vi "7.vi"() -> ()   [LabVIEW 2017]
uses:
  <vilib>/Waveform/WDTFileIO.llb/ Write Waveform to File.vi
  <vilib>/Waveform/WDTFileIO.llb/Read Waveform from File.vi
  <vilib>/Analysis/NI_AALBase.lvlib
panel:
  out "数组":dbl[](array[numeric])
  out "波形图":waveform(dbl)(graph)
  in  "cycles":dbl=1.0 caption="周期" format="%0.2f"
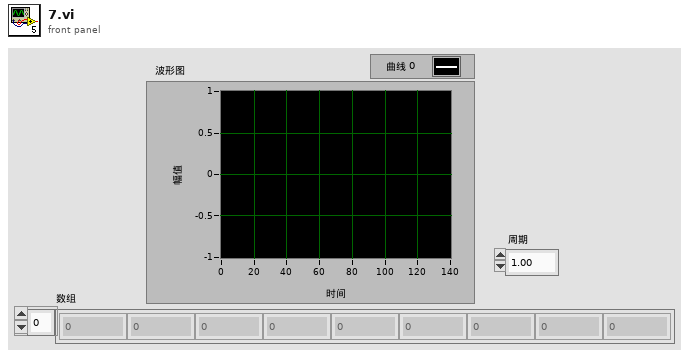
[diagram p1: front panel]
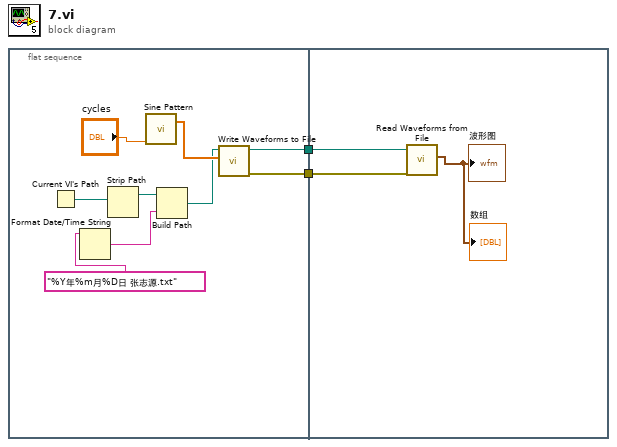
[diagram p0: block diagram]
diagram:
  n1 = flat-sequence {
    tunnel: [w4] -> w2
    tunnel: [w3] -> w1
    tunnel: w2 -> [w14]
    tunnel: w1 -> [w13]
    frame #0 {
      n2 = Current VI's Path() -> (path=w10:path)
      n3 = Format Date/Time String(time format string (%c)="%Y年%m月%D日 张志源.txt" ("时间格式字符串(%c)")) -> (date/time string=w8:string)  [unwired: 2 in]
      n4 = Strip Path(path=w10) -> (stripped path=w9:path)  [unwired: 1 out]
      n5 = call <vilib>:"Sine Pattern.vi"("cycles"="cycles") -> ("Sinusoidal Pattern"=w6:dbl[])  [unwired: 3 in, 1 out]
      n6 = Build Path(base path=w9, name or relative path=w8) -> (appended path=w5:path)
      n7 = call-poly <vilib>:"Write Waveforms to File.vi"("waveform"=w6, "file path (dialog if empty)"=w5) -> ("error out"=w3:errorcluster, "new file path (Not A Path if cancelled)"=w4:path)  [unwired: 8 in]
    }
    frame #1 {
      n8 = call-poly <vilib>:"Read Waveforms from File.vi"("error in (no error)"=w13, "file path (dialog if empty)"=w14) -> ("first waveform in record"=→"波形图" →"数组":waveform(dbl))  [unwired: 4 in, 3 out]
    }
  }
